vi "Interrogate_register.vi"(6 "Address override":i32, 8 "error in (no error)":errorcluster, 9 "UUT Index":i32, 10 "Register mutli-protocol location":T2={"General Parameter name"="", "MODBUS Register"=0, "Profibus"={"Friendly name"="", "PA"={"Slot"=0, "Index"=0}, "DP"={"Slot"=0, "Index"=0}, "Tag"=""}, "Fieldbus"={"Parameter name"="", "Fieldbus Block"="", "Fieldbus Tag"=""}, "data type"=enum."float", "DeviceNET"={"ClassId"=102, "InstanceId"=1, "AttributeId"=12}, "Cluster"={"address"=0, "Mode"=0}, "Length"=0} {"Cluster"."Mode" items=["None", "MODBUS", "HART", "Profibus DP", "Profibus PA", "Fieldbus", "DeviceNET"]}, 11 "DeviceNET in":refnum<class "DeviceNET.lvclass">) -> (0 "error out":errorcluster, 1 "Parameter name":string, 2 "output":sgl, 3 "DeviceNET out":refnum<class "DeviceNET.lvclass">, 4 "output cluster":T1)   [LabVIEW 2016, in "DeviceNET.lvclass"]
uses:
  DeviceNET.lvclass
  Typedef/comm_variable_definition.ctl
  Typedef/Comm_mode_and_address_type.ctl
  Typedef/Comm_mode_type_combo.ctl
  DeviceNET.lvclass/DeviceNET.ctl
  Protocol Class/Protocol.lvclass
  <vilib>/DeviceNet/DeviceNetLIB.lvlib
panel:
  out "cycle time (s)":dbl
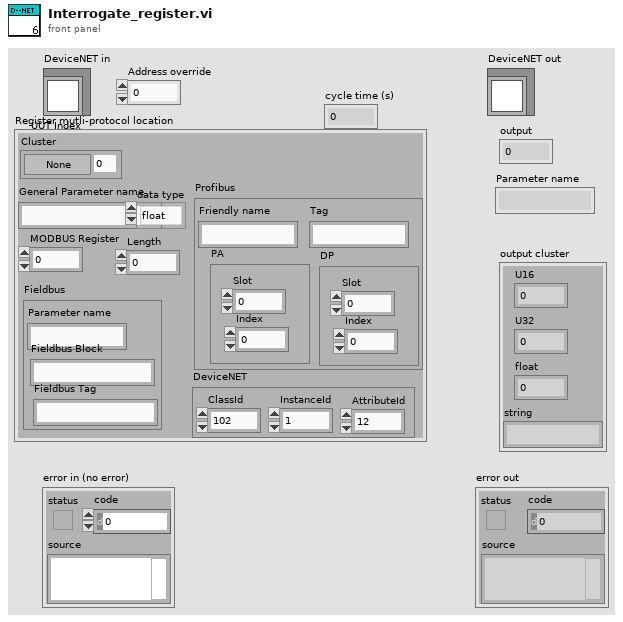
[diagram p1: front panel]
types:
  T1 = cluster{"U16":u16, "U32":u32, "float":sgl, "string":string}
  T2 = typedef "comm_variable_definition.ctl" = cluster{"General Parameter name":string, "MODBUS Register":i32, "Profibus":cluster{"Friendly name":string, "PA":cluster{"Slot":i32, "Index":i32}, "DP":cluster{"Slot":i32, "Index":i32}, "Tag":string}, "Fieldbus":cluster{"Parameter name":string, "Fieldbus Block":string, "Fieldbus Tag":string}, "data type":enum16{"float", "UINT", "UINT32", "STRING"}, "DeviceNET":cluster{"ClassId":u16, "InstanceId":u16, "AttributeId":u8}, "Cluster":T3, "Length":i32}
  T3 = typedef "Comm_mode_and_address_type.ctl" = cluster{"address":i32, "Mode":T4}
  T4 = typedef "Comm_mode_type_combo.ctl" = u16
  T5 = enum16{"BOOL (8[TF])", "SINT (I8)", "INT (I16)", "DINT (I32)", "USINT (U8)", "UINT (U16)", "UDINT (U32)", "REAL (SGL)", "LREAL (DBL)", "SHORT_STRING (abc)", "STRING (abc)"}
  T6 = cluster{"Device Address":i32, "Switch index":i32}[]
  T7 = enum16{"dnet0", "dnet1", "dnet2", "dnet3", "dnet4", "dnet5", "dnet6", "dnet7", "dnet8", "dnet9", "dnet10", "dnet11", "dnet12", "dnet13", "dnet14", "dnet15", "dnet16", "dnet17", "dnet18", "dnet19", "dnet20", "dnet21", "dnet22", "dnet23", "dnet24", "dnet25", "dnet26", "dnet27", "dnet28", "dnet29", "dnet30", "dnet31"}
  T8 = typedef "DeviceNetLIB.lvlib/xobjhandle.ctl" = u32
  T9 = cluster{"Device Address":i32, "Switch index":i32}
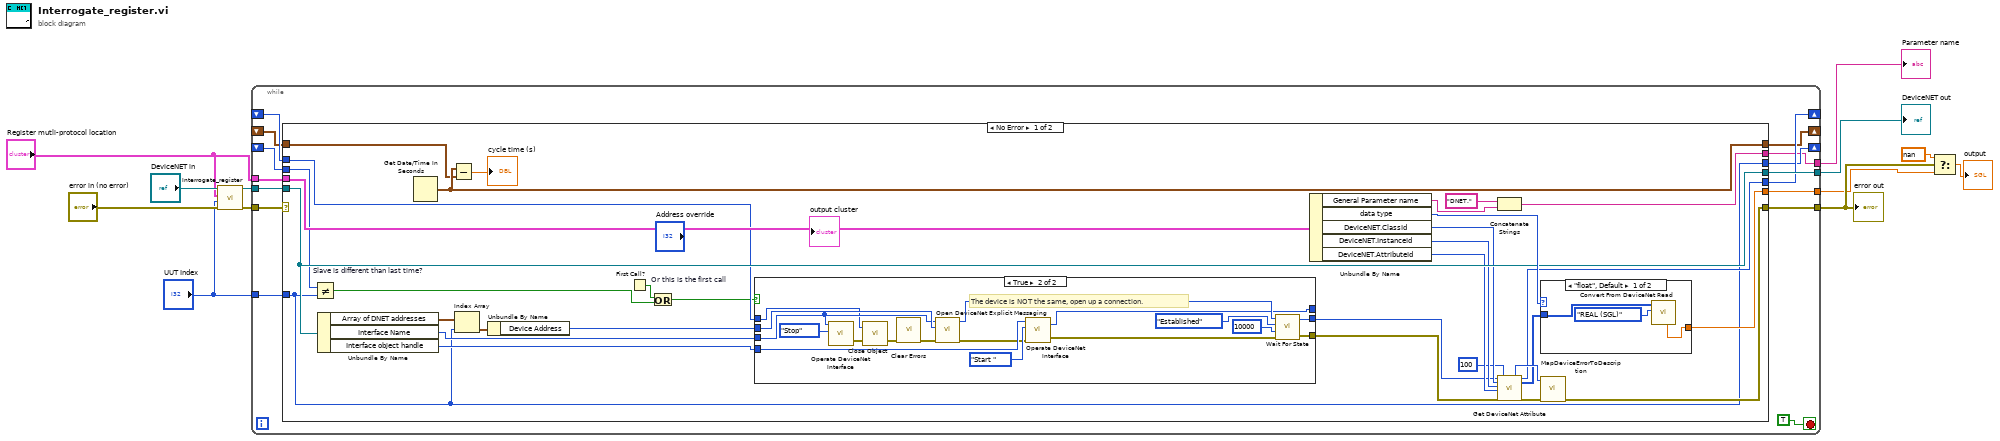
[diagram p0: block diagram]
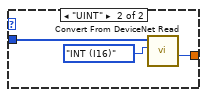
[diagram p3: hidden frame]
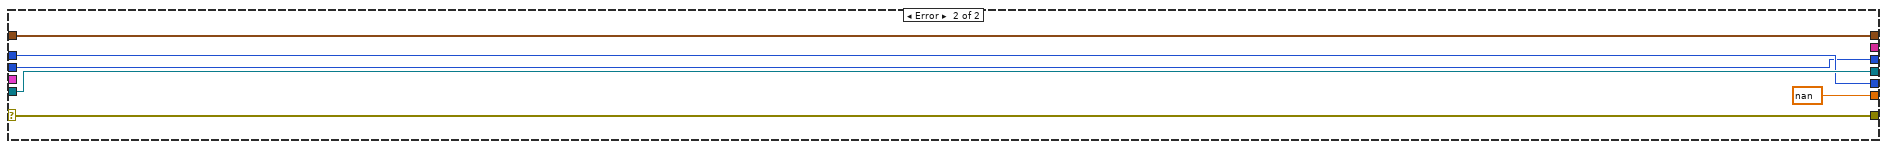
[diagram p4: hidden frame]
diagram:
  n1 = call-parent "Interrogate_register.vi"("error in (no error)"="error in (no error)", "UUT Index"="UUT Index", "Register mutli-protocol location"="Register mutli-protocol location", "Protocol in"="DeviceNET in") -> ("error out"=w10:errorcluster, "Protocol out"=w9:refnum<class "DeviceNET.lvclass">)  [unwired: 3 in, 3 out]
  n2 = while {
    tunnel: w10 -> [w27]
    tunnel: w9 -> [w26]
    tunnel: "Register mutli-protocol location" -> [w25]
    tunnel: "UUT Index" -> [w24]
    tunnel: [w23] -> w6
    tunnel: [w22] -> w5
    tunnel: [w21] -> w4
    shift-right: [w16] -> _
    shift-left: _ -> [w19]
    shift-right: [w18] -> _
    shift-left: _ -> [w17]
    shift-right: [w15] -> _
    shift-left: _ -> [w14]
    tunnel: [w13] -> w1
    stop <- TRUE stop-if-true
    n3 = case shown="No Error" w27 {
      selector: w27 -> [_ w90]
      tunnel: w25 -> [w59 _]
      tunnel: [w50 sgl nan ("type single")] -> w21
      tunnel: [w43 w90] -> w22
      tunnel: w24 -> [w33 _]
      tunnel: w26 -> [w57 w88]
      tunnel: [w57 w88] -> w23
      tunnel: w19 -> [w48 w86]
      tunnel: [w42 w87] -> w18
      tunnel: w17 -> [w45 w87]
      tunnel: [w33 w86] -> w16
      tunnel: [w37 w85] -> w15
      tunnel: w14 -> [w36 w85]
      tunnel: [w28 _] -> w13
      frame No Error {
        n4 = Not Equal? "Slave is different than last time?"(x=w48, y=w33) -> (x != y?=w46:bool)
        n5 = Unbundle By Name(w57) -> ("Array of DNET addresses"=w34:T6, "Interface Name"=w56:T7, "Interface object handle"=w40:T8)
        n6 = Get Date/Time In Seconds() -> (seconds since 1Jan1904=w37:timestamp)
        n7 = Subtract(x=w37, y=w36) -> (x-y=→"cycle time (s)":dbl)
        n8 = Index Array(array=w34, index=w33) -> (element=w32:T9)
        n9 = Unbundle By Name(w32) -> ("Device Address"=w31:i32)
        n10 = First Call?() -> (First Call?: T/F=w38:bool)
        n11 = Or "Or this is the first call"(x=w38, y=w46) -> (x .or. y?=w39:bool)
        n12 = case shown="True" w39 {
          tunnel: w56 -> [_ w64]
          tunnel: w40 -> [w60 w77]
          tunnel: [w61 w71] -> w41
          tunnel: [w60 w70] -> _
          tunnel: w31 -> [_ w69]
          tunnel: w45 -> [w61 w63]
          tunnel: [_ w62] -> w44
          frame False {
          }
          frame True {
            # "The device is NOT the same, open up a connection."
            n13 = call <vilib>:"Operate DeviceNet Interface.vi"("operation code (Start)"=enum16{"Start ", "Stop", "Active", "Idle"}."Stop", "object handle in"=w64) -> ("error out"=w67:errorcluster)  [unwired: 2 in, 1 out]
            n14 = call <vilib>:"Close Object.vi"("error in (no error)"=w67, "object handle in"=w63) -> ("error out"=w66:errorcluster)  [unwired: 1 in]
            n15 = call <vilib>:"Clear Errors.vi"("error in (no error)"=w66) -> ("error out"=w65:errorcluster)  [unwired: 5 in, 1 out]
            n16 = call <vilib>:"Open DeviceNet Explicit Messaging.vi"("error in (no error)"=w65, "device MAC ID"=w69, "interface name"=w64) -> ("error out"=w76:errorcluster, "object handle out"=w74:T8)  [unwired: 3 in]
            n17 = call <vilib>:"Operate DeviceNet Interface.vi"("error in (no error)"=w76, "operation code (Start)"=enum16{"Start ", "Stop", "Active", "Idle"}."Start ", "object handle in"=w77) -> ("error out"=w75:errorcluster, "object  handle out"=w70:T8)  [unwired: 1 in]
            n18 = call <vilib>:"Wait For State.vi"("error in (no error)"=w75, "timeout (0 ms)"=u32 10000, "desired state (Read Avail)"=enum16{"Read Avail", "Established"}."Established", "object handle in"=w74) -> ("error out"=w62:errorcluster, "object handle out"=w71:T8)  [unwired: 1 out]
          }
        }
        n19 = Unbundle By Name(w59) -> ("General Parameter name"=w29:string, "data type"=w58:enum16{"float", "UINT", "UINT32", "STRING"}, "DeviceNET.ClassId"=w55:u16, "DeviceNET.InstanceId"=w54:u16, "DeviceNET.AttributeId"=w53:u8)
        n20 = Concatenate Strings("DNET." ("Protocol name"), w29) -> (w28:string)
        n21 = call <vilib>:"Get DeviceNet Attribute.vi"("object handle in"=w41, "class ID (0)"=w55, "instance ID (0)"=w54, "attribute ID (0)"=w53, "error in (no error)"=w44, "timeout (100 ms)"=u32 100) -> ("device error"=w52:u16, "object handle out"=w42:T8, "attribute data"=w49:u8[], "error out"=w51:errorcluster)  [unwired: 9 in, 1 out]
        n22 = case shown="\"float\", Default" w58 {
          tunnel: [w79 w82] -> w50
          tunnel: w49 -> [w80 w83]
          frame "float", Default {
            n23 = call <vilib>:"Convert From DeviceNet Read.vi"("DeviceNet type (BOOL)"=T5."REAL (SGL)", "DeviceNet data in (0)"=w80) -> ("DBL/SGL out"=w79:dbl)  [unwired: 4 in, 5 out]
          }
          frame "UINT" {
            n24 = call <vilib>:"Convert From DeviceNet Read.vi"("DeviceNet type (BOOL)"=T5."INT (I16)", "DeviceNet data in (0)"=w83) -> ("I32/I16/I8 out"=w82:i32)  [unwired: 4 in, 5 out]
          }
        }
        n25 = call "MapDeviceErrorToDescription.vi"("error in"=w51, "device error"=w52) -> ("error out"=w43:errorcluster)  [unwired: 8 in, 1 out]
      }
      frame Error {
      }
    }
  }
  "error out" <- w5
  "DeviceNET out" <- w6
  "Parameter name" <- w1
  n26 = Select(t=nan, s=w5, f=w4) -> (s? t:f=→"output":dbl)
